vi "输入合法性检查.vi"(2 "被检查名称":string, 3 "合法名称集合":string[](array[string])) -> (0 "合法名称":string, 1 "输入有效":bool)   [LabVIEW 2013]
doc: "这个VI将被检查的名称与合法名称集合中的元素进行比较，如果被检查的名称与合法名称集合中的某一个元素的名称相同，则输入有效置1，并返回合法名称集合中的元素名称。\n例如：\n被检查名称可以是GV2，如何合法名称集合中存在GV这一项，则输入有效置1，且返回合法名称GV。否则将返回空字符串。"
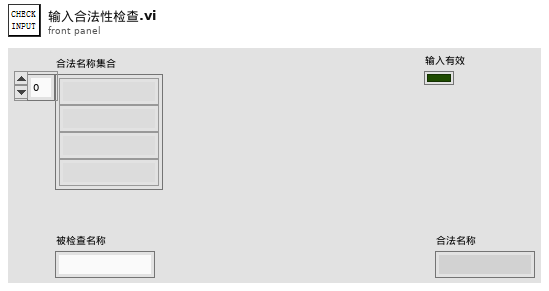
[diagram p1: front panel]
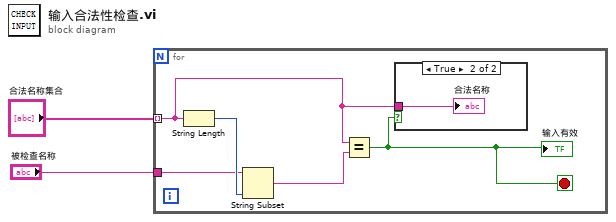
[diagram p0: block diagram]
diagram:
  n1 = for {
    tunnel: "合法名称集合" -> [w3] mode=indexing
    tunnel: "被检查名称" -> [w6]
    stop <- w4 stop-if-true
    n2 = String Length(string=w3) -> (length=w7:i32)
    n3 = String Subset(string=w6, length (rest)=w7) -> (substring=w5:string)  [unwired: 1 in]
    n4 = Equal?(x=w3, y=w5) -> (x = y?=w4:bool)
    "输入有效" <- w4
    n5 = case shown="True" w4 {
      tunnel: w3 -> [_ w8]
      frame False {
      }
      frame True {
        "合法名称" <- w8
      }
    }
  }
